vi "Doc_Builder_New_Report.vi"() -> (3 "NI_report out":refnum<class "NI_report.lvclass">)   [LabVIEW 2019]
uses:
  <vilib>/Utility/NIReport.llb/NI_report.lvclass
  <vilib>/Utility/NIReport.llb/Report Type.ctl
  <vilib>/Utility/NIReport.llb/NI_ReportGenerationCore.lvlib
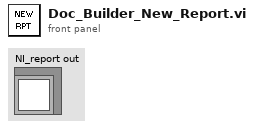
[diagram p1: front panel]
types:
  T1 = typedef "NI_ReportGenerationCore.lvlib/Report Type.ctl" = enum16{"HTML", "Word", "Excel"}
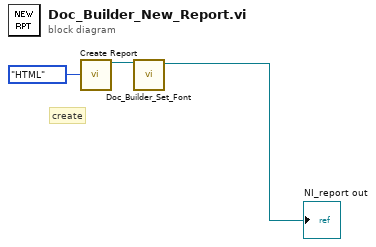
[diagram p0: block diagram]
diagram:
  # "create"
  n1 = call <vilib>:"Create Report.vi"("report type"=Report_Type."HTML") -> ("report out"=w1:refnum<class "NI_report.lvclass">)  [unwired: 13 in, 1 out]
  n2 = call "Doc_Builder_Set_Font.vi"("NI_report in"=w1) -> ("NI_report out"=→"NI_report out":refnum<class "NI_report.lvclass">)  [unwired: 10 in]
